vi "2 - MQTT_Q - Engine.vi"() -> ()   [LabVIEW 2015]
uses:
  source/MQTT_Q.lvclass
panel:
  out "Current Temperature":dbl
  out "Waveform Chart":dbl(graph)
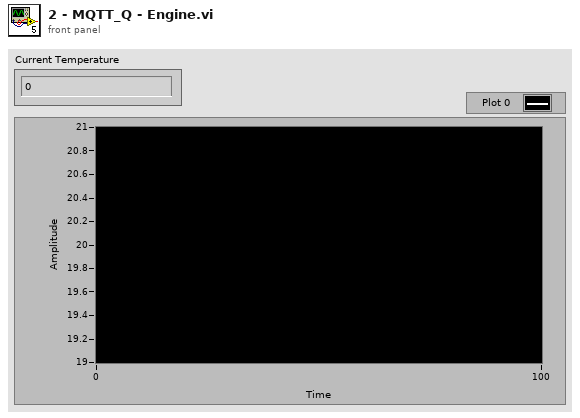
[diagram p1: front panel]
types:
  T1 = cluster{"IP address":string, "Port":u16, "Client ID":string}
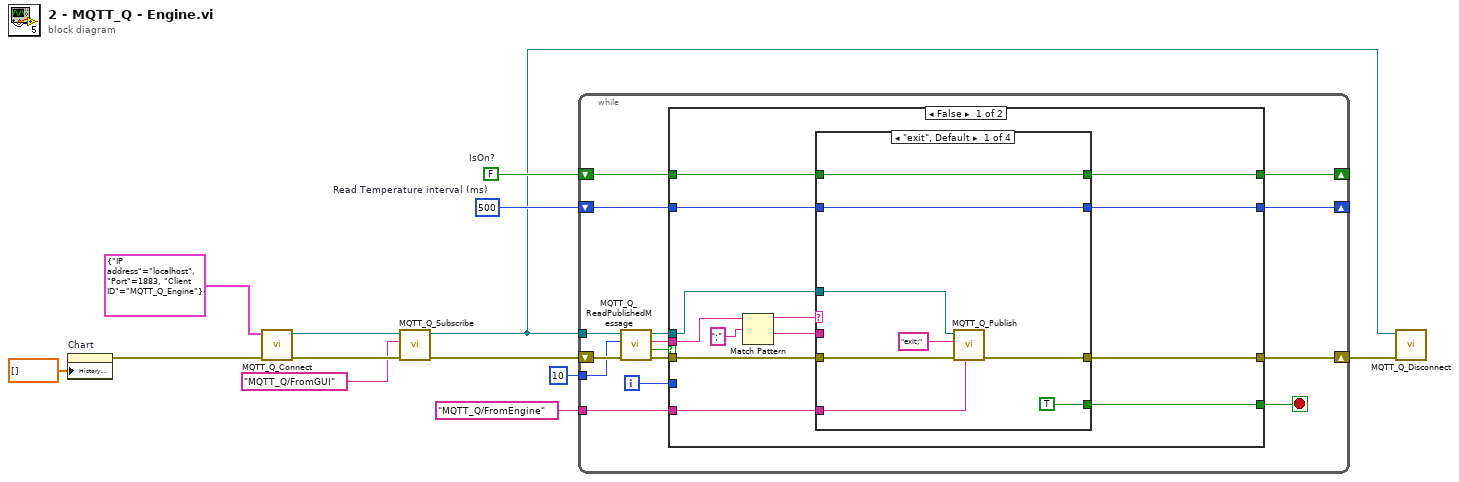
[diagram p0: block diagram]
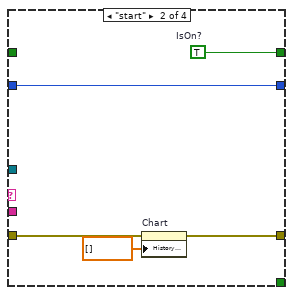
[diagram p2: hidden frame]
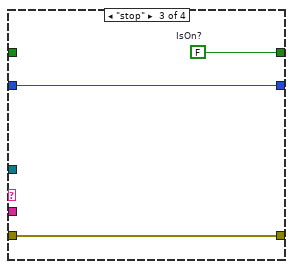
[diagram p3: hidden frame]
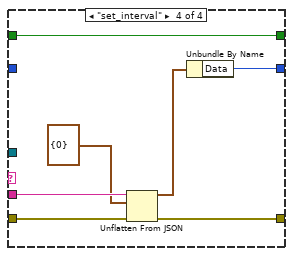
[diagram p4: hidden frame]
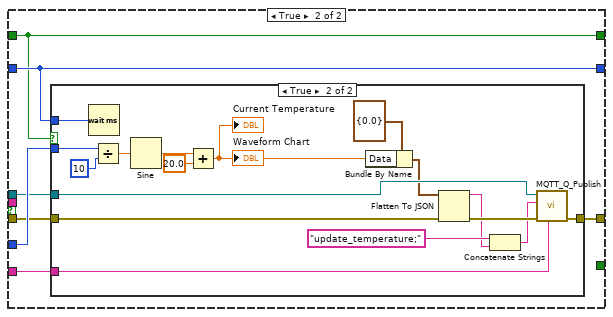
[diagram p5: hidden frame]
diagram:
  w11 = u32 500  # Read Temperature interval (ms)
  w12 = FALSE  # IsOn?
  n1 = property on="Chart" class="WFChart (strict)"("History Data"=dbl[] []) -> (error out=w9:errorcluster)  [unwired: 2 in, 1 out]
  n2 = call "MQTT_Q_Connect.vi"("error in (no error)"=w9, "MQTT Broker & Client ID"=T1 {"IP address"="localhost", "Port"=1883, "Client ID"="MQTT_Q_Engine"}) -> ("error out"=w6:errorcluster, "MQTT_Q Out"=w4:refnum<class "MQTT_Q.lvclass">)  [unwired: 8 in]
  n3 = call "MQTT_Q_Subscribe.vi"("error in (no error)"=w6, "Topic"="MQTT_Q/FromGUI", "MQTT_Q In"=w4) -> ("error out"=w5:errorcluster, "MQTT_Q Out"=w3:refnum<class "MQTT_Q.lvclass">)  [unwired: 6 in, 1 out]
  n4 = while {
    shift-right: [w24] -> w8
    shift-left: w5 -> [w27]
    tunnel: w3 -> [w23]
    shift-right: [w20] -> _
    shift-left: w12 -> [w17]
    shift-right: [w18] -> _
    shift-left: w11 -> [w19]
    tunnel: 10 ("timeout in ms (-1)") -> [w16]
    tunnel: "MQTT_Q/FromEngine" ("Topic") -> [w14]
    i -> [w28]
    stop <- w21 stop-if-true
    n5 = call "MQTT_Q_ReadPublishedMessage.vi"("error in (no error)"=w27, "timeout ms (25000)"=w16, "MQTT_Q In"=w23) -> ("error out"=w26:errorcluster, "TimedOut"=w25:bool, "Message"=w22:string, "MQTT_Q Out"=w15:refnum<class "MQTT_Q.lvclass">)  [unwired: 4 in, 1 out]
    n6 = case shown="False" w25 {
      tunnel: w28 -> [_ w71]
      tunnel: w26 -> [w33 w68]
      tunnel: [w40 w67] -> w24
      tunnel: w22 -> [w34 _]
      tunnel: [w41 _] -> w21
      tunnel: [w39 w69] -> w20
      tunnel: w19 -> [w38 w70]
      tunnel: [w37 w70] -> w18
      tunnel: w17 -> [w36 w69]
      tunnel: w15 -> [w29 w66]
      tunnel: w14 -> [w30 w65]
      frame False {
        n7 = Match Pattern(string=w34, regular expression=";") -> (before substring=w32:string, after substring=w31:string)  [unwired: 1 in, 2 out]
        n8 = case shown="\"exit\", Default" w32 {
          tunnel: [TRUE _ _ _] -> w41
          tunnel: w33 -> [w46 w53 w57 w62]
          tunnel: [w45 w52 w57 w61] -> w40
          tunnel: [w48 w51 w56 w64] -> w39
          tunnel: w38 -> [w47 w50 w55 _]
          tunnel: [w47 w50 w55 w58] -> w37
          tunnel: w36 -> [w48 _ _ w64]
          tunnel: w31 -> [_ _ _ w63]
          tunnel: w30 -> [w44 _ _ _]
          tunnel: w29 -> [w43 _ _ _]
          frame "exit", Default {
            n9 = call "MQTT_Q_Publish.vi"("Topic"=w44, "error in"=w46, "Message"="exit;", "MQTT_Q In"=w43) -> ("error out"=w45:errorcluster)  [unwired: 6 in, 1 out]
          }
          frame "start" {
            w51 = TRUE  # IsOn?
            n10 = property on="Chart" class="WFChart (strict)"(error in=w53, "History Data"=dbl[] []) -> (error out=w52:errorcluster)  [unwired: 1 in, 1 out]
          }
          frame "stop" {
            w56 = FALSE  # IsOn?
          }
          frame "set_interval" {
            n11 = Unflatten From JSON(JSON string=w63, type and defaults=cluster{"Data":u32} {"Data"=0}, error in (no error)=w62) -> (value=w59:cluster{"Data":u32}, error out=w61:errorcluster)  [unwired: 4 in]
            n12 = Unbundle By Name(w59) -> ("Data"=w58:u32)
          }
        }
      }
      frame True {
        n13 = case shown="True" w69 {
          tunnel: w71 -> [_ w88]
          tunnel: w70 -> [_ w84]
          tunnel: w68 -> [w72 w81]
          tunnel: [w72 w83] -> w67
          tunnel: w66 -> [_ w82]
          tunnel: w65 -> [_ w73]
          frame False {
          }
          frame True {
            n14 = Wait (ms)(milliseconds to wait=w84) -> ()  [unwired: 1 out]
            n15 = Divide(x=w88, y=10) -> (x/y=w89:dbl)
            n16 = Sine(x=w89) -> (sin(x)=w86:dbl)
            n17 = Add(x=w86, y=20.0) -> (x+y=w77:dbl)
            "Waveform Chart" <- w77
            "Current Temperature" <- w77
            n18 = Bundle By Name(cluster=cluster{"Data":dbl} {"Data"=0.0}, "Data"=w77) -> (w78:cluster{"Data":dbl})
            n19 = Flatten To JSON(anything=w78, error in (no error)=w81) -> (JSON string=w75:string, 11:w80:errorcluster)  [unwired: 1 in]
            n20 = Concatenate Strings("update_temperature;" ("Cmd"), w75) -> (w74:string)
            n21 = call "MQTT_Q_Publish.vi"("Topic"=w73, "error in"=w80, "Message"=w74, "MQTT_Q In"=w82) -> ("error out"=w83:errorcluster)  [unwired: 6 in, 1 out]
          }
        }
      }
    }
  }
  n22 = call "MQTT_Q_Disconnect.vi"("error in (no error)"=w8, "MQTT_Q In"=w3) -> ()  [unwired: 9 in, 1 out]
